vi "PigeonSensorReadings.vi"(1 "Reset Yaw":bool) -> (0 "Yaw (deg)":dbl format="%#_13g")   [LabVIEW 2018]
uses:
  refnums.vi
  <vilib>/Rock Robotics/WPI/ThirdParty/Phoenix-LabVIEW/Pigeon IMU/CTRE_PigeonIMU_GetYPR.vi
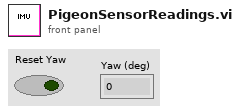
[diagram p1: front panel]
types:
  T1 = typedef "CTRE_PigeonIMU_DeviceRef.ctl" = cluster{"DeviceStatus":errorcluster, "Device Number":u8, "Type":T2, "Device ID":u32, "Handle":u64, "UsageFrame":u32, "Library Path":path}
  T2 = typedef "CTRE_PigeonIMU_ConnectionType.ctl" = u32
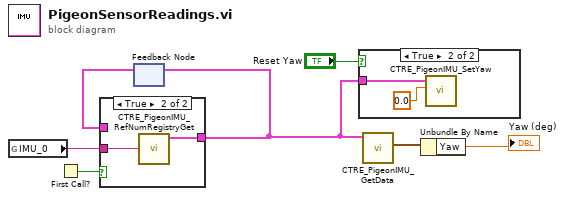
[diagram p0: block diagram]
diagram:
  n1 = global read "refnums.vi" "IMU_0"() -> (w2:string)
  n2 = First Call?() -> (First Call?: T/F=w4:bool)
  n3 = feedback #1() -> (w3:T1)  [unwired: 1 in]
  n4 = case shown="True" w4 {
    tunnel: [w8 w9] -> w1
    tunnel: w3 -> [w8 _]
    tunnel: w2 -> [_ w10]
    frame False {
    }
    frame True {
      n5 = call <vilib>:"CTRE_PigeonIMU_RefNumRegistryGet.vi"("refnum name"=w10) -> ("PigeonIMUDevRef"=w9:T1)  [unwired: 9 in, 1 out]
    }
  }
  n6 = feedback-in #1(w1) -> ()
  n7 = case shown="True" "Reset Yaw" {
    tunnel: w1 -> [_ w12]
    frame False {
    }
    frame True {
      n8 = call <vilib>:"CTRE_PigeonIMU_SetYaw.vi"("Value"=0.0, "PigeonIMUDevRef"=w12) -> ()  [unwired: 8 in, 2 out]
    }
  }
  n9 = call-poly <vilib>:"CTRE_PigeonIMU_GetData.vi"("PigeonIMUDevRef"=w1) -> ("Yaw Pitch Roll"=w7:cluster{"Yaw":dbl, "Pitch":dbl, "Roll":dbl})  [unwired: 8 in, 2 out]
  n10 = Unbundle By Name(w7) -> ("Yaw"=→"Yaw (deg)":dbl)
